vi "conv_7seg.vi"(3 "Numeric":i32) -> (0 "Boolean 2":bool, 1 "Boolean1":bool, 2 "Boolean 3":bool, 4 "Boolean 4":bool, 5 "Boolean 5":bool, 6 "Boolean 6":bool, 7 "Boolean 7":bool)   [LabVIEW 2010]
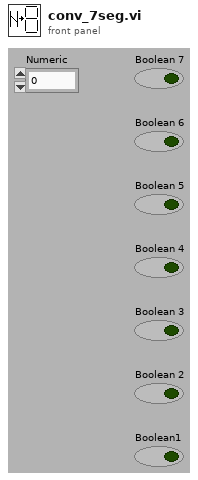
[diagram p1: front panel]
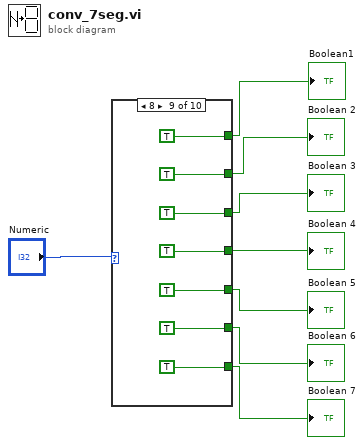
[diagram p0: block diagram]
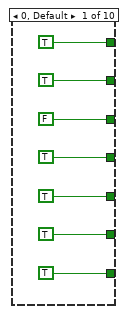
[diagram p2: hidden frame]
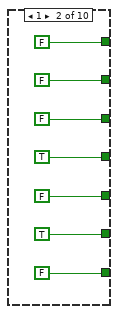
[diagram p3: hidden frame]
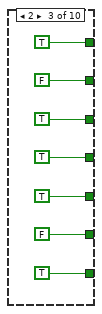
[diagram p4: hidden frame]
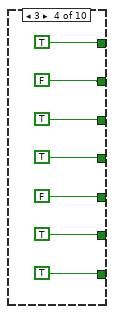
[diagram p5: hidden frame]
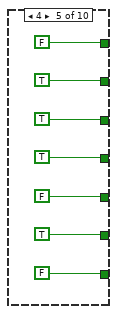
[diagram p6: hidden frame]
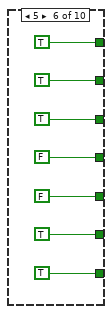
[diagram p7: hidden frame]
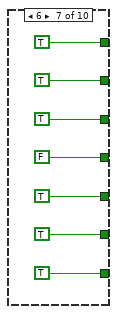
[diagram p8: hidden frame]
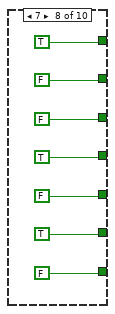
[diagram p9: hidden frame]
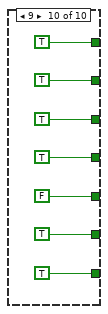
[diagram p10: hidden frame]
diagram:
  n1 = case shown="8" "Numeric" {
    tunnel: [TRUE FALSE TRUE TRUE FALSE TRUE TRUE TRUE TRUE TRUE] -> w7
    tunnel: [TRUE FALSE FALSE FALSE TRUE TRUE TRUE FALSE TRUE TRUE] -> w6
    tunnel: [FALSE FALSE TRUE TRUE TRUE TRUE TRUE FALSE TRUE TRUE] -> w5
    tunnel: [TRUE TRUE TRUE TRUE TRUE FALSE FALSE TRUE TRUE TRUE] -> w4
    tunnel: [TRUE FALSE TRUE FALSE FALSE FALSE TRUE FALSE TRUE FALSE] -> w3
    tunnel: [TRUE TRUE FALSE TRUE TRUE TRUE TRUE TRUE TRUE TRUE] -> w2
    tunnel: [TRUE FALSE TRUE TRUE FALSE TRUE TRUE FALSE TRUE TRUE] -> w1
    frame 0, Default {
    }
    frame 1 {
    }
    frame 2 {
    }
    frame 3 {
    }
    frame 4 {
    }
    frame 5 {
    }
    frame 6 {
    }
    frame 7 {
    }
    frame 8 {
    }
    frame 9 {
    }
  }
  "Boolean1" <- w7
  "Boolean 2" <- w6
  "Boolean 3" <- w5
  "Boolean 4" <- w4
  "Boolean 5" <- w3
  "Boolean 6" <- w2
  "Boolean 7" <- w1
